vi "SLL DE AI Engine.vi"(8 "error in (no error)":errorcluster, 11 "Delay (ms)":u32=100) -> (0 "error out":errorcluster)   [LabVIEW 2013]
doc: "Copyright © 2005, Soliton Technologies.\nAll rights reserved."
uses:
  Controls/SLL DE DAQ Engine Options.ctl
  Controls/SLL DE DAQ Engine Channel Types.ctl
  Controls/SLL DE AI Global Options.ctl
  Controls/SLL DE DAQ Global Options.ctl
  Controls/SLL DE DAQ Global Elements.ctl
  <vilib>/DAQmx/read.llb/DAQmx Read (Analog 2D DBL NChan NSamp).vi
  <vilib>/Analysis/baseanly.llb/Mean (DBL).vi
  <vilib>/DAQmx/miscellaneous.llb/DAQmx Fill In Error Info.vi
  <vilib>/Analysis/NI_AALBase.lvlib
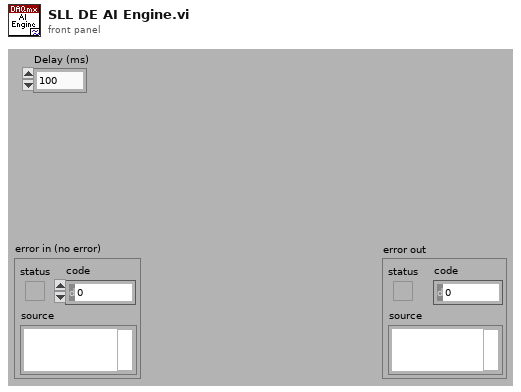
[diagram p1: front panel]
types:
  T1 = typedef "SLL DE DAQ Engine Options.ctl" = enum16{">Init", ">Safe Mode", ">Poll", ">Error", ">Exit", ">Restart", ">DI", ">DO", ">AI", ">AO", ">Start Task", ">Stop Task"}
  T2 = typedef "SLL DE DAQ Global Options.ctl" = enum16{"Init", "Write 1", "Read 1", "Write Array", "Read Array", "Clear"}
  T3 = typedef "SLL DE AI Global Options.ctl" = enum16{"Init", "Write Line", "Write Array", "Read Line", "Read Array", "Read Full Status", "Write Full Status"}
  T4 = typedef "SLL DE DAQ Engine Channel Types.ctl" = enum16{"Analog Input", "Analog Output", "Digital Input", "Digital Output"}
  T5 = cluster{"Array of Tasks":refnum<k21>[], "Channel Order":i32[], "AI Data":dbl[]}
  T6 = typedef "SLL DE DAQ Global Elements.ctl" = enum16{"AI Error", "AO Error", "DI Error", "DO Error", "AI Restart", "DI Restart", "AI Running", "AO Running", "DI Running", "DO Running", "DAQ Exit?"}
  T7 = enum16{"Left Button", "Center Button", "Right Button", "Window Close"}
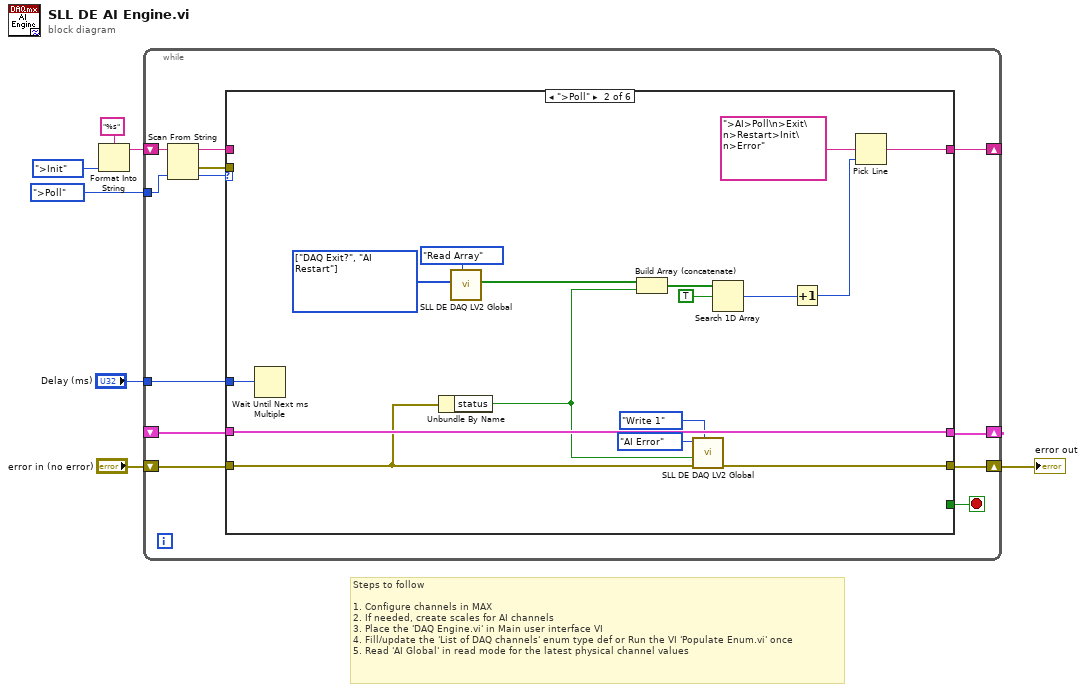
[diagram p0: block diagram]
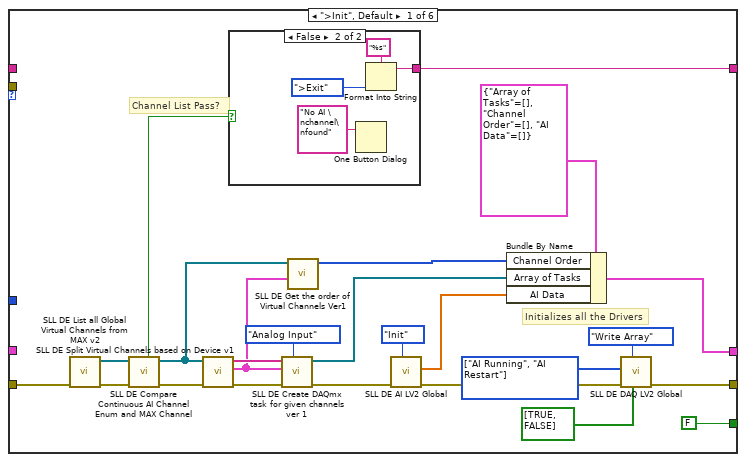
[diagram p2: hidden frame]
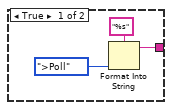
[diagram p3: hidden frame]
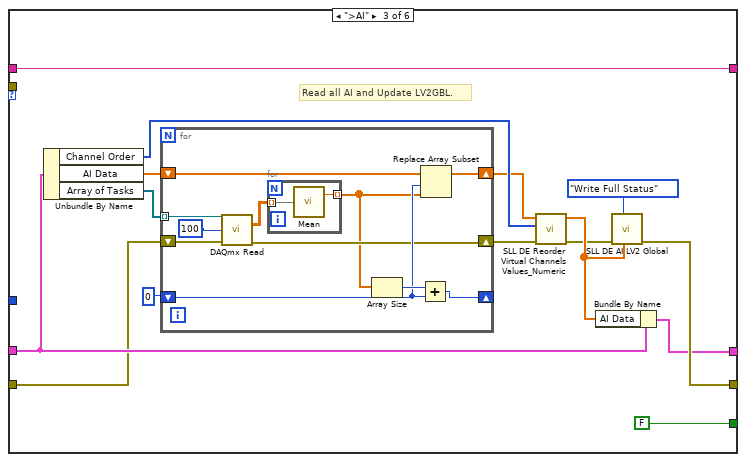
[diagram p4: hidden frame]
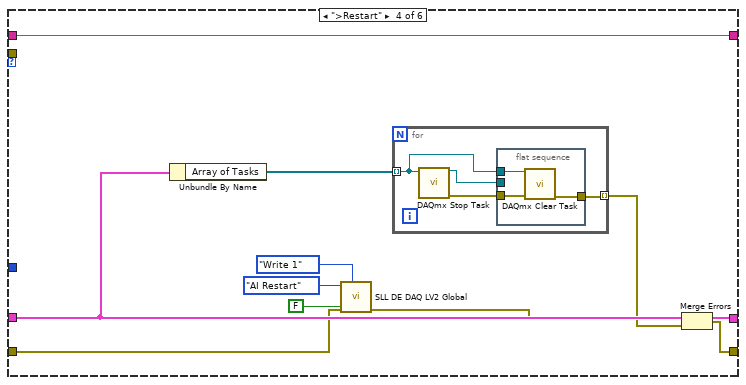
[diagram p5: hidden frame]
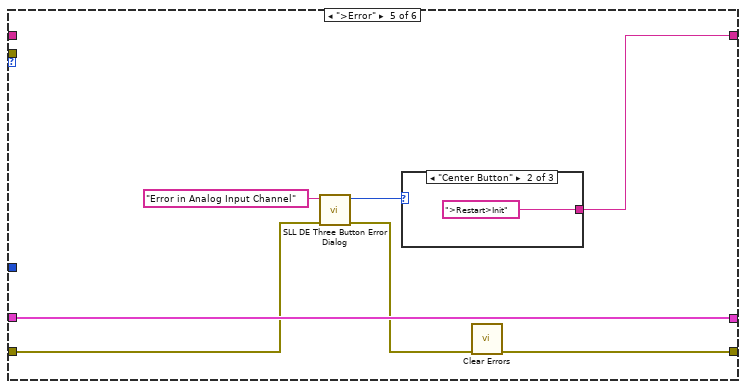
[diagram p6: hidden frame]
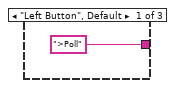
[diagram p7: hidden frame]
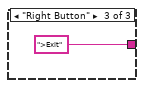
[diagram p8: hidden frame]
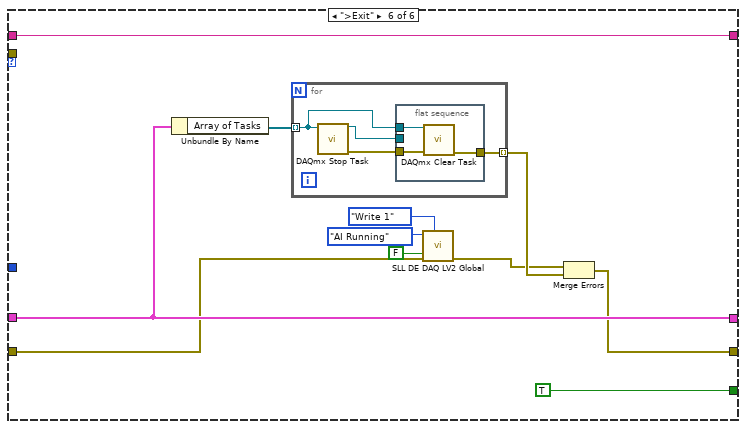
[diagram p9: hidden frame]
diagram:
  # "Steps to follow\n\n1.\tConfigure channels in MAX\n2.\tIf needed, create scales for AI channels\n3.\tPlace the 'DAQ Engine.vi' in Main user interface VI\n4.\tFill/update the 'List of DAQ channels' enum type def or Run the VI 'Populate Enum.vi' once\n5.\tRead 'AI Global' in read mode for the latest physical channel values"
  n1 = Format Into String(format string="%s", SLL_DE_DAQ_Engine_Options.">Init" ("DAQ Options")) -> (resulting string=w3:string)  [unwired: 2 in, 1 out]
  n2 = while {
    shift-right: [w18] -> w6
    shift-left: "error in (no error)" -> [w19]
    shift-right: [w17] -> _
    shift-left: _ -> [w16]
    shift-right: [w12] -> _
    shift-left: w3 -> [w15]
    tunnel: "Delay (ms)" -> [w10]
    tunnel: SLL_DE_DAQ_Engine_Options.">Poll" ("DAQ Options") -> [w8]
    stop <- w11 stop-if-true
    n3 = Scan From String(input string=w15, default 1=w8) -> (remaining string=w14:string, error out=w13:errorcluster, output 1=w9:T1)  [unwired: 3 in, 1 out]
    n4 = case shown="\">Poll\"" w9 {
      tunnel: w19 -> [w20 w56 w68 w99 w113 w122]
      tunnel: [w36 w55 w79 w95 w115 w127] -> w18
      tunnel: [w43 w66 w71 w104 w118 w130] -> w17
      tunnel: w16 -> [_ w66 w72 w104 w118 w130]
      tunnel: w14 -> [_ _ w81 w98 _ w132]
      tunnel: w13 -> [_ _ _ _ _ _]
      tunnel: [w39 w60 w81 w98 w114 w132] -> w12
      tunnel: [FALSE _ FALSE _ _ TRUE] -> w11
      tunnel: w10 -> [_ w59 _ _ _ _]
      frame ">Init", Default {
        w35 = T6[] [enum."AI Running", enum."AI Restart"] items=["AI Error", "AO Error", "DI Error", "DO Error", "AI Restart", "DI Restart", "AI Running", "AO Running", "DI Running", "DO Running", "DAQ Exit?"] ("Elements Array")
        # "Channel List Pass?"
        # "Initializes all the Drivers"
        n5 = call "SLL DE List all Global Virtual Channels from MAX v2.vi"("error in (no error)"=w20) -> ("error out"=w25:errorcluster, "Analog Input"=w22:refnum<k21>[])  [unwired: 4 in, 5 out]
        n6 = call "SLL DE Compare Continuous AI Channel Enum and MAX Channel.vi"("error in (no error)"=w25, "Analog Input Channels"=w22) -> ("error out"=w24:errorcluster, "Channels Out"=w23:refnum<k21>[], "Pass?"=w21:bool)  [unwired: 7 in]
        n7 = call "SLL DE Split Virtual Channels based on Device v1.vi"("error in (no error)"=w24, "GlobalChans"=w23) -> ("error out"=w31:errorcluster, "Channel Array"=w27:cluster{"Device Channel List":string[]}[], "Devices Names"=w32:string[])  [unwired: 7 in]
        n8 = case shown="False" w21 {
          tunnel: [w44 w48] -> w39
          frame True {
            n9 = Format Into String(format string="%s", SLL_DE_DAQ_Engine_Options.">Poll" ("DAQ Options")) -> (resulting string=w44:string)  [unwired: 2 in, 1 out]
          }
          frame False {
            n10 = One Button Dialog(message="No AI \nchannel\nfound") -> ()  [unwired: 1 in, 1 out]
            n11 = Format Into String(format string="%s", SLL_DE_DAQ_Engine_Options.">Exit" ("DAQ Options")) -> (resulting string=w48:string)  [unwired: 2 in, 1 out]
          }
        }
        n12 = call "SLL DE Create DAQmx task for given channels ver 1.vi"("Channel Type"=SLL_DE_DAQ_Engine_Channel_Types."Analog Input", "error in (no error)"=w31, "Channel Array"=w27, "Devices Names"=w32) -> ("error out"=w28:errorcluster, "Array of Tasks"=w30:refnum<k21>[])  [unwired: 6 in]
        n13 = call "SLL DE Get the order of Virtual Channels Ver1.vi"("Channel Array"=w27, "Virtial Channels Info"=w23) -> ("Channel Order"=w29:i32[])  [unwired: 8 in, 1 out]
        n14 = call "SLL DE AI LV2 Global.vi"("AI Option"=SLL_DE_AI_Global_Options."Init", "error in (no error)"=w28) -> ("error out"=w37:errorcluster, "Analog Input Array Value"=w42:dbl[])  [unwired: 7 in, 1 out]
        n15 = Bundle By Name(cluster=T5 {"Array of Tasks"=[], "Channel Order"=[], "AI Data"=[]} ("Data Cluster"), "Channel Order"=w29, "Array of Tasks"=w30, "AI Data"=w42) -> (w43:T5)
        n16 = call "SLL DE DAQ LV2 Global.vi"("Status Array In"=bool[] [TRUE, FALSE], "Option"=SLL_DE_DAQ_Global_Options."Write Array", "error in (no error)"=w37, "Elements Array"=w35) -> ("error out"=w36:errorcluster)  [unwired: 5 in, 2 out]
      }
      frame ">Poll" {
        w52 = T6[] [enum."DAQ Exit?", enum."AI Restart"] items=["AI Error", "AO Error", "DI Error", "DO Error", "AI Restart", "DI Restart", "AI Running", "AO Running", "DI Running", "DO Running", "DAQ Exit?"] ("Elements Array")
        n17 = Wait Until Next ms Multiple(millisecond multiple=w59) -> ()  [unwired: 1 out]
        n18 = Unbundle By Name(w56) -> ("status"=w54:bool)
        n19 = call "SLL DE DAQ LV2 Global.vi"("Option"=SLL_DE_DAQ_Global_Options."Read Array", "Elements Array"=w52) -> ("Status Array Out"=w51:bool[])  [unwired: 7 in, 2 out]
        n20 = Build Array (concatenate)(w51, w54) -> (w64:bool[])
        n21 = call "SLL DE DAQ LV2 Global.vi"("Option"=SLL_DE_DAQ_Global_Options."Write 1", "error in (no error)"=w56, "Status In"=w54, "Element"=SLL_DE_DAQ_Global_Elements."AI Error") -> ("error out"=w55:errorcluster)  [unwired: 5 in, 2 out]
        n22 = Search 1D Array(1D array=w64, element=TRUE) -> (index of element=w62:i32)  [unwired: 1 in]
        n23 = Increment(x=w62) -> (x+1=w61:i32)
        n24 = Pick Line(multi-line string=">AI>Poll\n>Exit\n>Restart>Init\n>Error", line index=w61) -> (output string=w60:string)  [unwired: 1 in]
      }
      frame ">AI" {
        # "Read all AI and Update LV2GBL."
        n25 = Unbundle By Name(w72) -> ("Channel Order"=w74:i32[], "AI Data"=w76:dbl[], "Array of Tasks"=w77:refnum<k21>[])
        n26 = for {
          tunnel: w77 -> [w87] mode=indexing
          shift-right: [w91] -> w73
          shift-left: w76 -> [w92]
          shift-right: [w88] -> _
          shift-left: 0 -> [w89]
          shift-right: [w85] -> w67
          shift-left: w68 -> [w86]
          n27 = call-poly <vilib>:"DAQmx Read.vi"("task/channels in"=w87, "number of samples per channel"=100, "error in"=w86) -> ("data"=w83:dbl[][], "error out"=w85:errorcluster)  [unwired: 10 in, 1 out]
          n28 = for {
            tunnel: w83 -> [w94] mode=indexing
            tunnel: [w93] -> w82 mode=indexing
            n29 = call-poly <vilib>:"Mean.vi"("X"=w94) -> ("mean"=w93:dbl)  [unwired: 1 out]
          }
          n30 = Array Size(array=w82) -> (size(s)=w90:i32)
          n31 = Add(x=w90, y=w89) -> (x+y=w88:i32)
          n32 = Replace Array Subset(array=w92, new element=w82, index=w89) -> (w91:dbl[])
        }
        n33 = call "SLL DE Reorder Virtual Channels Values_Numeric.vi"("error in (no error)"=w67, "Channel Order"=w74, "Disordered DI Data"=w73) -> ("error out"=w69:errorcluster, "Ordered DI Data"=w70:dbl[])  [unwired: 7 in]
        n34 = Bundle By Name(cluster=w72, "AI Data"=w70) -> (w71:T5)
        n35 = call "SLL DE AI LV2 Global.vi"("AI value Array"=w70, "AI Option"=SLL_DE_AI_Global_Options."Write Full Status", "error in (no error)"=w69) -> ("error out"=w79:errorcluster)  [unwired: 6 in, 2 out]
      }
      frame ">Restart" {
        n36 = Unbundle By Name(w104) -> ("Array of Tasks"=w103:refnum<k21>[])
        n37 = call "SLL DE DAQ LV2 Global.vi"("Option"=SLL_DE_DAQ_Global_Options."Write 1", "error in (no error)"=w99, "Status In"=FALSE, "Element"=SLL_DE_DAQ_Global_Elements."AI Restart") -> ("error out"=w97:errorcluster)  [unwired: 5 in, 2 out]
        n38 = for {
          tunnel: w103 -> [w108] mode=indexing
          tunnel: [w105] -> w96 mode=indexing
          n39 = call <vilib>:"DAQmx Stop Task.vi"("task/channels in"=w108) -> ("task out"=w107:refnum<k21>, "error out"=w106:errorcluster)  [unwired: 13 in]
          n40 = flat-sequence {
            tunnel: w108 -> [w111]
            tunnel: w107 -> [_]
            tunnel: w106 -> [w110]
            tunnel: [w109] -> w105
            frame #0 {
              n41 = call <vilib>:"DAQmx Clear Task.vi"("task in"=w111, "error in"=w110) -> ("error out"=w109:errorcluster)  [unwired: 13 in]
            }
          }
        }
        n42 = Merge Errors(w97, w96) -> (w95:errorcluster)
      }
      frame ">Error" {
        n43 = call "SLL DE Three Button Error Dialog.vi"("Error In"=w113, "Window Title"="Error in Analog Input Channel") -> ("Error Out"=w112:errorcluster, "Which Button?"=w116:T7)  [unwired: 8 in]
        n44 = case shown="\"Center Button\"" w116 {
          tunnel: [">Poll" ("Window Title") ">Restart>Init" ("Window Title") ">Exit" ("Window Title")] -> w114
          frame "Left Button", Default {
          }
          frame "Center Button" {
          }
          frame "Right Button" {
          }
        }
        n45 = call <vilib>:"Clear Errors.vi"("error in (no error)"=w112) -> ("error out"=w115:errorcluster)  [unwired: 6 in]
      }
      frame ">Exit" {
        n46 = Unbundle By Name(w130) -> ("Array of Tasks"=w129:refnum<k21>[])
        n47 = for {
          tunnel: w129 -> [w136] mode=indexing
          tunnel: [w133] -> w128 mode=indexing
          n48 = call <vilib>:"DAQmx Stop Task.vi"("task/channels in"=w136) -> ("task out"=w135:refnum<k21>, "error out"=w134:errorcluster)  [unwired: 13 in]
          n49 = flat-sequence {
            tunnel: w136 -> [w139]
            tunnel: w135 -> [_]
            tunnel: w134 -> [w137]
            tunnel: [w138] -> w133
            frame #0 {
              n50 = call <vilib>:"DAQmx Clear Task.vi"("task in"=w139, "error in"=w137) -> ("error out"=w138:errorcluster)  [unwired: 13 in]
            }
          }
        }
        n51 = call "SLL DE DAQ LV2 Global.vi"("Option"=SLL_DE_DAQ_Global_Options."Write 1", "error in (no error)"=w122, "Status In"=FALSE, "Element"=SLL_DE_DAQ_Global_Elements."AI Running") -> ("error out"=w125:errorcluster)  [unwired: 5 in, 2 out]
        n52 = Merge Errors(w125, w128) -> (w127:errorcluster)
      }
    }
  }
  "error out" <- w6
